vi "Random 0-9999 String.vi"() -> (0 "random 0-999 String string":string)   [LabVIEW 2014]
doc: "Concatenate random number 0-9999 to end of input String."
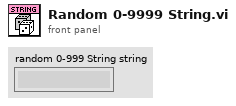
[diagram p1: front panel]
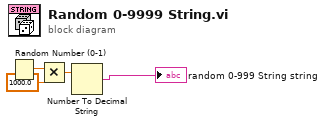
[diagram p0: block diagram]
diagram:
  n1 = Random Number (0-1)() -> (number: 0 to 1=w2:dbl)
  n2 = Multiply(x=w2, y=1000.0) -> (x*y=w4:dbl)
  n3 = Number To Decimal String(number=w4) -> (decimal integer string=→"random 0-999 String string":string)  [unwired: 1 in]
